vi "Close.vi"(8 "error in (no error)":errorcluster, 11 "bt_Blackboard in":refnum<class "Blackboard.lvclass">) -> (0 "error out":errorcluster, 3 "bt_Blackboard out":refnum<class "Blackboard.lvclass">)   [LabVIEW 2021, in "Blackboard.lvclass"]
uses:
  Blackboard.lvclass
  Blackboard.lvclass/Blackboard.ctl
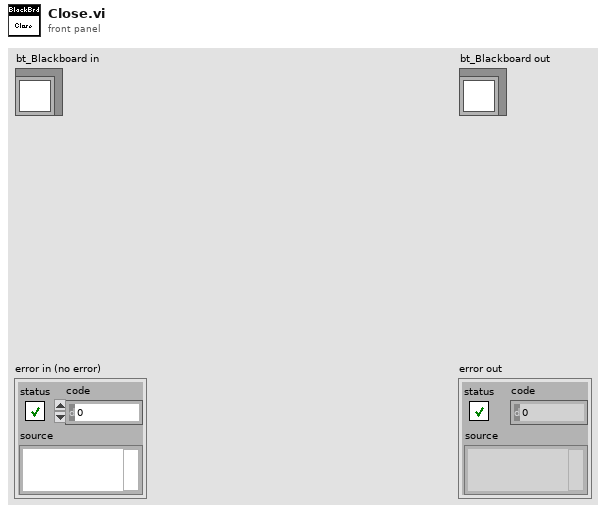
[diagram p1: front panel]
types:
  T1 = typedef "Blackboard.lvclass/Data DVR Type.ctl" = cluster{"Tags":T2, "Status":refnum<data-value>, "Boolean":refnum<data-value>, "String":refnum<data-value>, "DBL":refnum<data-value>, "SGL":refnum<data-value>, "EXT":refnum<data-value>, "U8":refnum<data-value>, "U16":refnum<data-value>, "U32":refnum<data-value>, "U64":refnum<data-value>, "I8":refnum<data-value>, "I16":refnum<data-value>, "I32":refnum<data-value>, "I64":refnum<data-value>, "CDBL":refnum<data-value>, "CSGL":refnum<data-value>, "CEXT":refnum<data-value>, "Time":refnum<data-value>, "Variant":refnum<data-value>, "Waveform":refnum<data-value>}
  T2 = typedef "Blackboard.lvclass/Tags Map Type.ctl" = map{string, cluster{"Data Index":i32, "Status Index":i32}}
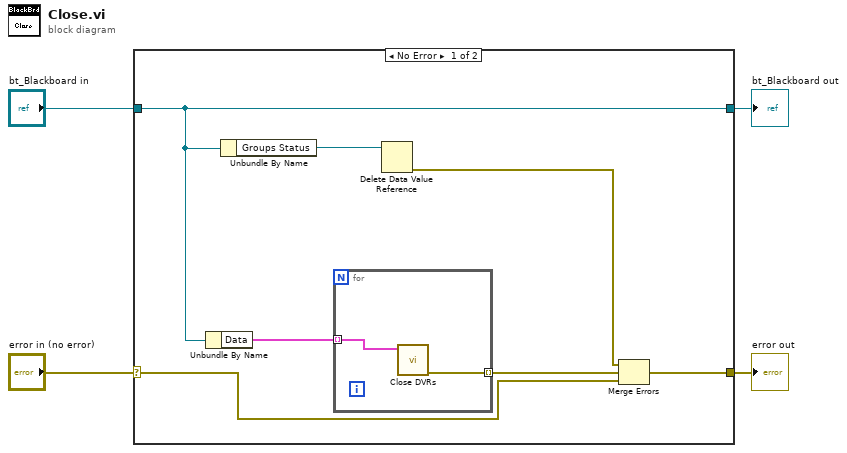
[diagram p0: block diagram]
diagram:
  n1 = case shown="No Error" "error in (no error)" {
    selector: "error in (no error)" -> [w8 w15]
    tunnel: [w9 w15] -> w3
    tunnel: [w6 w14] -> w1
    tunnel: "bt_Blackboard in" -> [w6 w14]
    frame No Error {
      n2 = Unbundle By Name(w6) -> ("Data"=w11:T1[])
      n3 = Unbundle By Name(w6) -> ("Groups Status"=w7:refnum<data-value>)
      n4 = for {
        tunnel: w11 -> [w13] mode=indexing
        tunnel: [w12] -> w10 mode=indexing
        n5 = call "Close DVRs.vi"("Data"=w13) -> ("error out"=w12:errorcluster)  [unwired: 10 in]
      }
      n6 = Delete Data Value Reference(data value reference=w7) -> (error out=w5:errorcluster)  [unwired: 1 in, 1 out]
      n7 = Merge Errors(w5, w10, w8) -> (w9:errorcluster)
    }
    frame Error {
    }
  }
  "error out" <- w3
  "bt_Blackboard out" <- w1
